vi "Dropable_DSA.vi"(0 "TF Out (CH B)":dbl, 1 "Cycle Specs":T2={"Cycles To Settle (M)"=5, "Cycles To Calculate (N)"=5}, 2 "Excitation Specs":T1={"Initial Frequency"=1.0, "Final Frequency"=100.0, "Number of Frequencies"=3, "Samping Time [s]"=0.001, "Amplitude [V]"=1.0, "Offset [V]"=0.5, "Freq Unit"=FALSE}, 5 "TF In (CH A)":dbl, 9 "START":bool, 11 "STOP":bool, 12 "Exist Porgram":bool) -> (4 "Disturbance":dbl, 6 "Bode Magnitude":cluster{dbl[], dbl[]}(graph)={[1.0, 1.2689610031679222, 1.6102620275609394, 2.043359717856942, 2.592943797404667, 3.2903445623126686, 4.1753189365604015, 5.298316906283708, 6.7233575364993365, 8.531678524172808, 10.826367338740546, 13.73823795883263, 17.43328822199988, 22.122162910704493, 28.072162039411772, 35.62247890262442, 45.20353656360243, 57.36152510448679, 72.7895384398315, 92.36708571873861, 117.21022975334806, 148.73521072935117, 188.73918221350976, 239.5026619987486, 303.9195382313198, 385.6620421163472, 489.3900918477494, 621.0169418915616, 788.0462815669912, 1000.0], [1.0018651131002922, 1.0016050465725763, 1.0010062349698785, 1.0002931137870483, 0.9991459144089636, 0.9972202532472595, 0.9944020144562293, 0.9903082002861369, 0.983855401702225, 0.9738705481650444, 0.9582906977613652, 0.9358034848813956, 0.9036393454169751, 0.857649976648417, 0.7964400088413218, 0.7217565791716765, 0.6359239660806931, 0.5476382842843324, 0.461415834347026, 0.38116988425483045, 0.3091314427820101, 0.2514928062528439, 0.20170891904461263, 0.15879614847289658, 0.127858110424497, 0.10171304349328705, 0.08081117825531599, 0.06376794604720305, 0.050469140870365095, 0.039745706120179934]}, 8 "Bode Phase":cluster{dbl[], dbl[]}(graph)={[1.0, 1.2689610031679222, 1.6102620275609394, 2.043359717856942, 2.592943797404667, 3.2903445623126686, 4.1753189365604015, 5.298316906283708, 6.7233575364993365, 8.531678524172808, 10.826367338740546, 13.73823795883263, 17.43328822199988, 22.122162910704493, 28.072162039411772, 35.62247890262442, 45.20353656360243, 57.36152510448679, 72.7895384398315, 92.36708571873861, 117.21022975334806, 148.73521072935117, 188.73918221350976, 239.5026619987486, 303.9195382313198, 385.6620421163472, 489.3900918477494, 621.0169418915616, 788.0462815669912, 1000.0], [-1.4001864556390353, -1.7425257743205063, -2.2774811113746067, -2.940300047591337, -3.797024621582645, -4.874740361894845, -6.244214499985965, -7.9488896703659435, -10.107416371370137, -12.8129960492024, -16.195047872218314, -20.2121008365249, -24.982209581081694, -30.62002310970157, -36.70295501035055, -43.18506539585506, -49.773026506300724, -56.0120451118291, -61.68921924132383, -66.61507141784128, -71.21117465500357, -75.07757805867544, -77.49128997241446, -81.82799122918105, -82.40583459630555, -84.09391534817092, -87.5421411007668, -88.23137376055858, -91.93060722680163, -98.46625820370649]}, 10 "Live Signals":cluster{"DSA Excitation":dbl, "output y(t)":dbl}(graph), 14 "Stopped":bool, 15 "Running":bool)   [LabVIEW 2017, in "DSA.lvlib"]
doc: "This program performs 3 tasks:\n\n A.) generates a swept sine wave over a specified number of logmartically spaced frequencies over a specified range,\n\n B.) outputs the swept sine wave point by point to a system and for each point output measues the system's response at two points\n\n C.) and using the two responses measured, calculates the bode magnitude and phase plots between the two points of the system.\n\nThis program is written as a state machine that itterates one time for every iteration of the loop that contains it.\n \nThe state is the current sample being measured. \nNOTE: Since we must excite the system before recording data, the current sample being measured is one less than the number of itterations the loop containing this subVI has run.\n\nTo perform these tasks, the following state machine does the following:\n\n INITIALIZATION \n\n When initalized, the state is set to 0 and the following are calculated:\n\n A.) a list of logmartically spaced frequencies to excite the system at, \n B.) the number of samples needed to be ignored in waiting for the excitation to settle for each frequency, \n C.) the number of samples needed to be measured in order to calculate the frequency response for each frequency,\n D.) and the total number of samples needed (total # of smaples ignored + total # of samples measured).\n\n < see (1) INITIALIZE THE DSA section in the block diagram >\n\n RUNNING\n\n When running, the following tasks are done:\n\n A.) The swept sine wave for the next sample to be measured is generated and output. \n This is done by generating:\n\n 1.) the ith point of the swept sine wave to excite the system\n 2.) the frequency of the sine wave for the current point\n 3.) and the index of the frequency within the list excitation frequencies that corresponds to the i+1 point's sine wave's frequency.\n\n < see (2A) GENERATE SWEPT SINE EXCITATIONS section in the block diagram >\n\n B.) Compare the current sample to:\n\n 1.) the current last sample to be ignored in the list of last samples to be ignored\n 2.) and the current last smaple taken before chaning frequencies in the list of sample taken before the frequency change.\n\n < see (2B) COLLECT DATA? section in the block diagram >\n\n C.) If the current sample:\n \n 1.) < the current last sample to be ignored:\n \n - do nothing.\n \n 2.) = the current last sample to be ignored and:\n\n\n a.) < the current sample taken before changing frequencies:\n \n - collect a sample on each channel and store it\n\n < see (2C) ANALYZE DATA section in the block diagram >\n\n b.) = the current sample taken before changing frequencies:\n\n i.) collect a sample on each channel and store it,\n ii.) with all the other samples stored for that excitation frequency, calculate the magnitude and phase for each channel,\n iii.) use the magnitude and phase for each channel to calculate the magnitude and phase between the two points in the system,\n iv.) and plot the magnitude and phase between those two points in the system on the bode plot for the frequency.\n \n < see (2D) VERIFY DATA & (2E) PLOT section in the block diagram >\n\nInputs: \n\n- Excitation Specs:\n\n - Initial Frequency: The lowest frequency of the frequency range which the DSA will measure the bode plot for. \n\n - Final Frequency: The highest frequency of the frequency range which the DSA will measure the bode plot for. \n\n - Frequency Units: Whether the frequecny range input is in Hz or rads/sec. \n \n - Number of Frequencies: The number of logmarithmically spaced frequencies to measure the bode plot for.\n\n - Sampling Time: The time step taking in between each measurement. Also equal to 1/(sampling rate)\n\n - Amplitude: Amplitude of desired swept sine excitation. \n\n - Offset: DC offset of swept sine excitation.\n\n- Cycle Specs:\n\n - Cycles to Settle: The number of cycles of the swept sine wave at each frequency to ignore to let the transcient response die out. \n\n - Cycles to Calculate: The number of cycles of the sept since wave at each frequency to measure in order to measure the bode plot.\n\n- Controls:\n\n - START: Tells the DSA to initalize and then start.\n\n - STOP: Tells the DSA to stop and set all analog outputs to zero.\n\n - EXIT PROGRAM: Tells LabVIEW to set all analog outputs to zero and exit the program.\n\n- Signals:\n\n - Analog In CH1: Response read by the A/D converter of the system at a given point to the swept sine excitation.\n\n - Analog In CH0: Response read by the A/D converter of the system at a given point to the swept sine excitation.\n\nOutputs:\n\n- Analog Out: Swept sine excitation wave sent to the D/A converter.\n\n- Running: Signal to show if the DSA is running.\n\n- Stopped: Signal to show if the DSA is stopped.\n\n- Bode Magnitude: The magnitude plot of the TF CH1/CH0.\n\n- Bode Phase: The phase plot of the TF CH1/CH0."
uses:
  DSA.lvlib
  <vilib>/Analysis/NI_AALPro.lvlib
panel:
  # "Dropable Dynamic Signal Analyzer"
  # "Magnitude"
  # "Dynamic Signal Analyzer"
  # "Controls"
  # "Signals"
  # "Phase"
  # "Excitation Frequencies"
  # "Frequency\nUnits"
  # "[Hz]"
  # "Excitation Magnitude"
  # "[rad/s]"
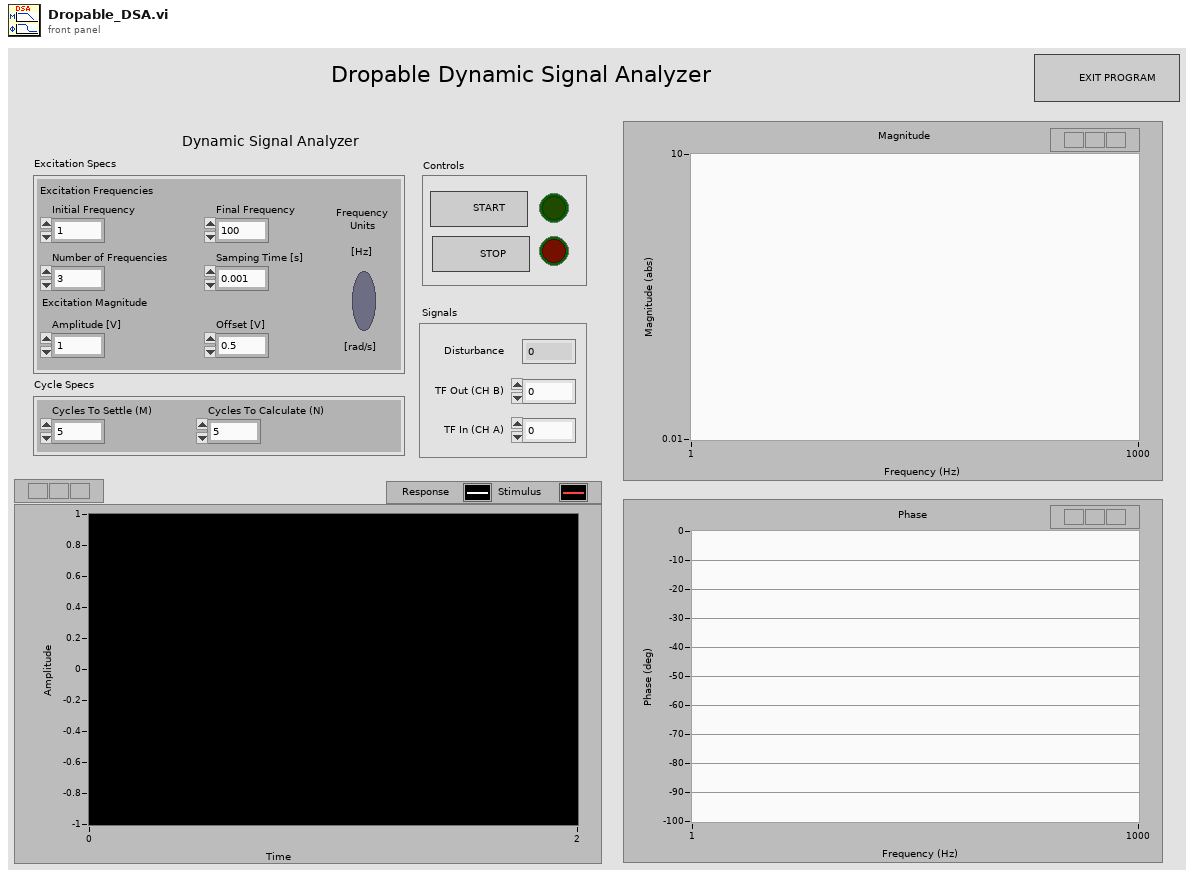
[diagram p1: front panel]
types:
  T1 = cluster{"Initial Frequency":dbl, "Final Frequency":dbl, "Number of Frequencies":i16, "Samping Time [s]":dbl, "Amplitude [V]":dbl, "Offset [V]":dbl, "Freq Unit":bool}
  T2 = cluster{"Cycles To Settle (M)":i16, "Cycles To Calculate (N)":i16}
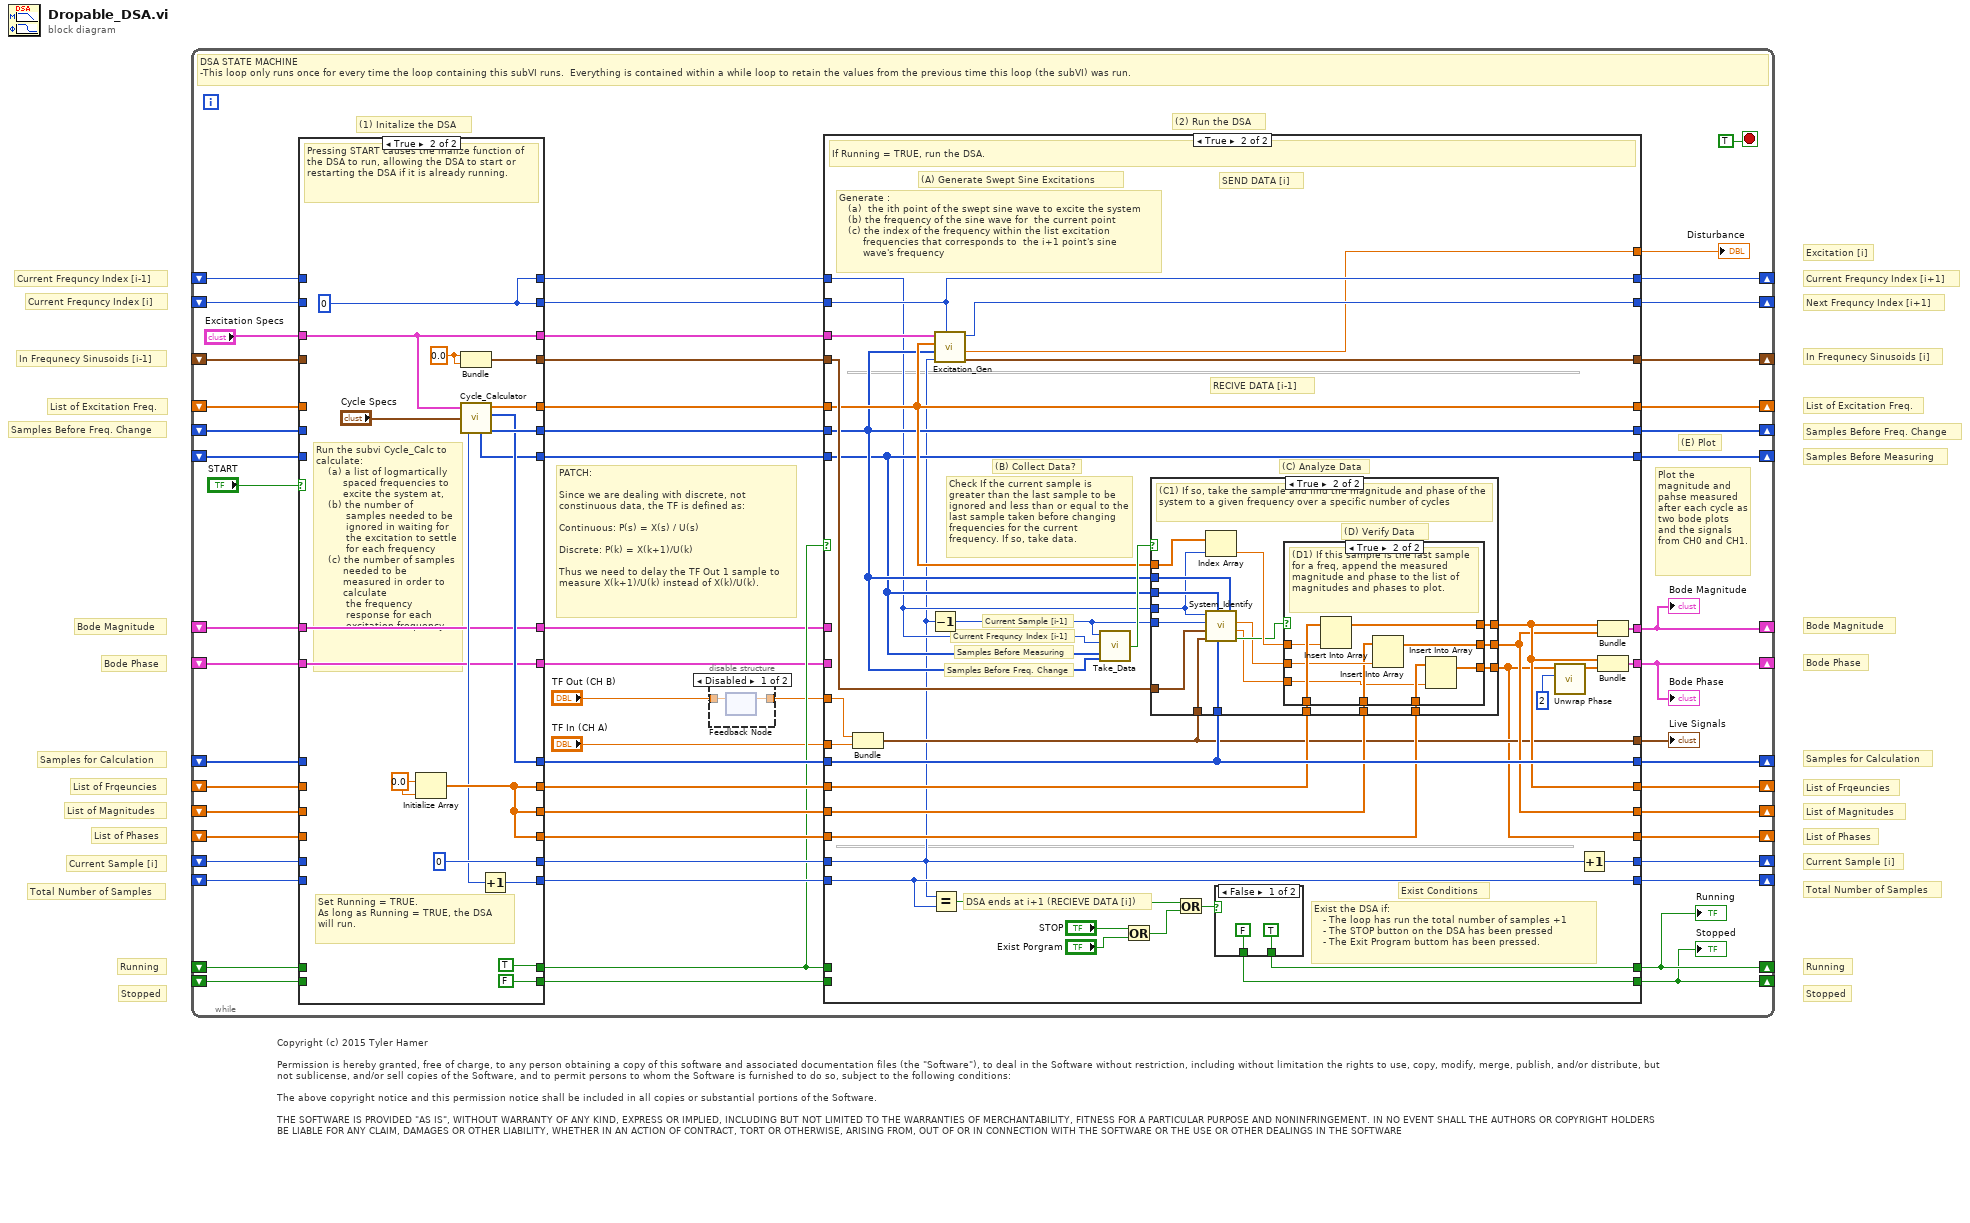
[diagram p0: block diagram]
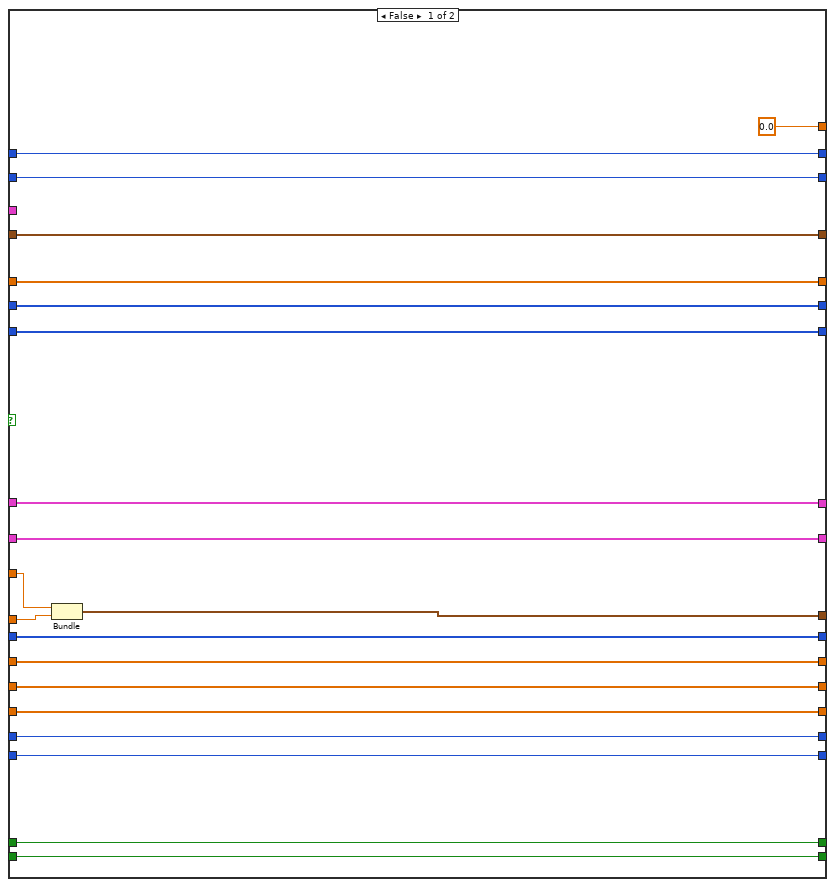
[diagram p4: hidden frame]
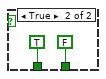
[diagram p5: hidden frame]
diagram:
  # "Copyright (c) 2015 Tyler Hamer\n\nPermission is hereby granted, free of charge, to any person obtaining a copy of this software and associated documentation files (the \"Software\"), to deal in the Software without restriction, including without limitation the rights to use, copy, modify, merge, publish, and/or distribute, but not sublicense, and/or sell copies of the Software, and to permit persons to whom the Software is furnished to do so, subject to the following conditions:\n\nThe above copyright notice and this permission notice shall be included in all copies or substantial portions of the Software.\n\nTHE SOFTWARE IS PROVIDED \"AS IS\", WITHOUT WARRANTY OF ANY KIND, EXPRESS OR IMPLIED, INCLUDING BUT NOT LIMITED TO THE WARRANTIES OF MERCHANTABILITY, FITNESS FOR A PARTICULAR PURPOSE AND NONINFRINGEMENT. IN NO EVENT SHALL THE AUTHORS OR COPYRIGHT HOLDERS BE LIABLE FOR ANY CLAIM, DAMAGES OR OTHER LIABILITY, WHETHER IN AN ACTION OF CONTRACT, TORT OR OTHERWISE, ARISING FROM, OUT OF OR IN CONNECTION WITH THE SOFTWARE OR THE USE OR OTHER DEALINGS IN THE SOFTWARE"
  # "Bode Phase"
  # "Bode Magnitude"
  # "Bode Phase"
  # "Bode Magnitude"
  # "Stopped"
  # "Running"
  # "Stopped"
  # "Running"
  # "Total Number of Samples"
  # "Total Number of Samples"
  # "List of Phases"
  # "List of Magnitudes"
  # "List of Frqeuncies"
  # "List of Phases"
  # "List of Magnitudes"
  # "List of Frqeuncies"
  # "Samples Before Measuring"
  # "Samples Before Freq. Change"
  # "Current Sample [i]"
  # "Samples for Calculation"
  # "Excitation [i]"
  # "List of Excitation Freq."
  # "In Frequnecy Sinusoids [i]"
  # "Next Frequncy Index [i+1]"
  # "Current Frequncy Index [i+1]"
  # "Samples for Calculation"
  # "Current Sample [i]"
  # "Samples Before Freq. Change"
  # "In Frequnecy Sinusoids [i-1]"
  # "Current Frequncy Index [i-1]"
  # "Current Frequncy Index [i]"
  # "List of Excitation Freq."
  n1 = while {
    shift-right: [w49] -> _
    shift-left: _ -> [w53]
    shift-right: [w51] -> _
    shift-left: _ -> [w52]
    shift-right: [w47] -> _
    shift-left: _ -> [w46]
    shift-right: [w40] -> _
    shift-left: _ -> [w50]
    shift-right: [w44] -> _
    shift-left: _ -> [w43]
    shift-right: [w37] -> _
    shift-left: _ -> [w36]
    shift-right: [w34] -> _
    shift-left: _ -> [w33]
    shift-right: [w31] -> _
    shift-left: _ -> [w30]
    shift-right: [w23] -> _
    shift-left: _ -> [w26]
    shift-right: [w22] -> _
    shift-left: _ -> [w25]
    shift-right: [w21] -> _
    shift-left: _ -> [w24]
    shift-right: [w18] -> _
    shift-left: _ -> [w17]
    shift-right: [w12] -> _
    shift-left: _ -> [w16]
    shift-right: [w11] -> _
    shift-left: _ -> [w13]
    shift-right: [w5] -> _
    shift-left: _ -> [w10]
    shift-right: [w4] -> _
    shift-left: _ -> [w9]
    stop <- TRUE stop-if-true
    # "PATCH:\n \nSince we are dealing with discrete, not constinuous data, the TF is defined as:\n \nContinuous: P(s) = X(s) / U(s) \n \nDiscrete: P(k) = X(k+1)/U(k)\n \nThus we need to delay the TF Out 1 sample to measure X(k+1)/U(k) instead of X(k)/U(k)."
    # "Plot the magnitude and pahse measured after each cycle as two bode plots and the signals from CH0 and CH1."
    # "(E) Plot"
    # "(2) Run the DSA"
    # "(1) Initalize the DSA"
    # "DSA STATE MACHINE \n-This loop only runs once for every time the loop containing this subVI runs.  Everything is contained within a while loop to retain the values from the previous time this loop (the subVI) was run."
    n2 = case shown="True" "START" {
      tunnel: "Excitation Specs" -> [w77 w94]
      tunnel: [w77 w94] -> w55
      tunnel: [w75 w93] -> w54
      tunnel: w53 -> [w75 _]
      tunnel: [w76 w91] -> w48
      tunnel: w52 -> [w76 _]
      tunnel: [w72 w92] -> w41
      tunnel: w50 -> [w72 _]
      tunnel: [w74 w91] -> w45
      tunnel: w46 -> [w74 _]
      tunnel: w43 -> [w73 _]
      tunnel: [w73 w89] -> w42
      tunnel: [w71 0] -> w39
      tunnel: w36 -> [w71 _]
      tunnel: [w70 w87] -> w35
      tunnel: w33 -> [w70 _]
      tunnel: [w69 w86] -> w32
      tunnel: w30 -> [w69 _]
      tunnel: [w68 w84] -> w29
      tunnel: [w67 w84] -> w28
      tunnel: [w66 w84] -> w27
      tunnel: w26 -> [w68 _]
      tunnel: w25 -> [w67 _]
      tunnel: w24 -> [w66 _]
      tunnel: [w65 w81] -> w19
      tunnel: w17 -> [w65 _]
      tunnel: w16 -> [w64 _]
      tunnel: [w64 TRUE] -> w15
      tunnel: [w63 FALSE] -> w14
      tunnel: w13 -> [w63 _]
      tunnel: w10 -> [w62 w79]
      tunnel: w9 -> [w61 w78]
      tunnel: [w62 w79] -> w8
      tunnel: [w61 w78] -> w7
      frame False {
      }
      frame True {
        w85 = 0.0
        w90 = 0.0
        w91 = 0
        # "Run the subvi Cycle_Calc to calculate: \n    (a) a list of logmartically \n         spaced frequencies to \n         excite the system at, \n    (b) the number of \n          samples needed to be \n          ignored in waiting for \n          the excitation to settle \n          for each frequency \n    (c) the number of samples \n         needed to be \n         measured in order to\n         calculate \n          the frequency   \n          response for each \n          excitation frequency."
        # "Set Running = TRUE.\nAs long as Running = TRUE, the DSA\nwill run."
        # "Pressing START causes the inalize function of the DSA to run, allowing the DSA to start or restarting the DSA if it is already running."
        n3 = Initialize Array(w85, w85) -> (w84:dbl[])
        n4 = Bundle(w90, w90) -> (w89:cluster{dbl, dbl})  [unwired: 1 in]
        n5 = call "Cycle_Calculator.vi"("Cycle Specs"="Cycle Specs", "Excitation Specs"=w94) -> ("Samples Before Frequency Change"=w92:i32[], "Samples Before Measuring"=w86:i32[], "Samples for Calculation"=w87:i32[], "Excitation Frequencies"=w93:dbl[], "Total Number of Samples"=w80:i32)  [unwired: 1 in, 1 out]
        n6 = Increment(x=w80) -> (x+1=w81:i32)
      }
    }
    n7 = disable-structure shown="Disabled" {
      disable-tunnel: "TF Out (CH B)" -> [w59 w60]
      disable-tunnel: [w58 w60] -> w2
      frame Disabled {
        n8 = feedback #1() -> (w58:dbl)  [unwired: 1 in]
        n9 = feedback-in #1(w59) -> ()
      }
      frame Enabled {
      }
    }
    n10 = case shown="True" w15 {
      tunnel: w55 -> [_ w151]
      tunnel: w54 -> [w115 w144]
      tunnel: [w114 w150] -> w51
      tunnel: [w115 w144] -> w49
      tunnel: w48 -> [w114 w149]
      tunnel: [w113 w149] -> w47
      tunnel: w45 -> [w113 w141]
      tunnel: [w112 w148] -> w44
      tunnel: w42 -> [w112 w145]
      tunnel: w41 -> [w111 w143]
      tunnel: [w111 w143] -> w40
      tunnel: w39 -> [w110 w119]
      tunnel: [w110 w147] -> w37
      tunnel: w35 -> [w109 w137]
      tunnel: [w109 w137] -> w34
      tunnel: w32 -> [w108 w142]
      tunnel: [w108 w142] -> w31
      tunnel: w2 -> [w99 w139]
      tunnel: "TF In (CH A)" -> [w98 w138]
      tunnel: w29 -> [w107 w136]
      tunnel: w28 -> [w106 w135]
      tunnel: w27 -> [w105 w134]
      tunnel: [w107 w133] -> w23
      tunnel: [w106 w132] -> w22
      tunnel: [w105 w118] -> w21
      tunnel: [0.0 w131] -> w20
      tunnel: w19 -> [w104 w123]
      tunnel: [w104 w123] -> w18
      tunnel: w15 -> [w103 _]
      tunnel: [w103 w125] -> w12
      tunnel: [w102 w124] -> w11
      tunnel: w14 -> [w102 _]
      tunnel: [w101 w121] -> w5
      tunnel: [w100 w120] -> w4
      tunnel: w8 -> [w101 _]
      tunnel: w7 -> [w100 _]
      tunnel: [w97 w122] -> w6
      frame False {
        n11 = Bundle("TF Out (CH B)"=w99, "TF In (CH A)"=w98) -> (w97:cluster{"TF Out (CH B)":dbl, "TF In (CH A)":dbl})  [unwired: 1 in]
      }
      frame True {
        # "(C) Analyze Data"
        # "Exist Conditions"
        # "Exist the DSA if:\n   - The loop has run the total number of samples +1\n   - The STOP button on the DSA has been pressed\n   - The Exit Program buttom has been pressed."
        # "DSA ends at i+1 (RECIEVE DATA [i])"
        # "SEND DATA [i]"
        # "RECIVE DATA [i-1]"
        # "Samples Before Freq. Change"
        # "Samples Before Measuring"
        # "Current Frequncy Index [i-1]"
        # "Current Sample [i-1]"
        # "(B) Collect Data?"
        # "Check If the current sample is greater than the last sample to be ignored and less than or equal to the last sample taken before changing frequencies for the current frequency. If so, take data."
        # "(A) Generate Swept Sine Excitations"
        # "Generate :\n   (a)  the ith point of the swept sine wave to excite the system\n   (b) the frequency of the sine wave for  the current point\n   (c) the index of the frequency within the list excitation \n        frequencies that corresponds to  the i+1 point's sine \n        wave's frequency"
        # "If Running = TRUE, run the DSA."
        n12 = Bundle("TF Out (CH B)"=w139, "TF In (CH A)"=w138) -> (w122:cluster{"TF Out (CH B)":dbl, "TF In (CH A)":dbl})  [unwired: 1 in]
        n13 = Decrement(x=w119) -> (x-1=w140:i32)
        n14 = Equal?(x=w119, y=w123) -> (x = y?=w130:bool)
        n15 = call "Excitation_Gen.vi"("Current Frequency Index"=w149, "Current Sample"=w119, "Samples Before Frequency Change"=w143, "Excitation Frequencies"=w144, "Excitation Specs"=w151) -> ("In Frequency Sinusoids"=w148:cluster{"cos(wt)":dbl, " sin(wt)":dbl}, "Excitation Sinusoid"=w131:dbl, "New Frequency Index"=w150:i32)  [unwired: 1 out]
        n16 = call "Take_Data.vi"("Samples Before Frequency Change"=w143, "Samples Before Measuring"=w142, "Current Frequency Index"=w141, "Current Sample"=w140) -> ("Take Data"=w146:bool)
        n17 = Or(x="STOP", y="Exist Porgram") -> (x .or. y?=w127:bool)
        n18 = case shown="True" w146 {
          tunnel: w145 -> [_ w172]
          tunnel: w122 -> [_ w176]
          tunnel: w140 -> [_ w175]
          tunnel: w141 -> [_ w169]
          tunnel: w142 -> [_ w174]
          tunnel: w143 -> [_ w173]
          tunnel: w144 -> [_ w171]
          tunnel: w137 -> [_ w170]
          tunnel: w136 -> [w158 w164]
          tunnel: w135 -> [w157 w163]
          tunnel: w134 -> [w156 w162]
          tunnel: [w158 w161] -> w133
          tunnel: [w157 w160] -> w132
          tunnel: [w156 w159] -> w118
          frame False {
            # "(C2) If not, ignore the current samples. Pass throught the list of measured magnitude and phases though."
          }
          frame True {
            # "(D) Verify Data"
            # "(C1) If so, take the sample and find the magnitude and phase of the system to a given frequency over a specific number of cycles"
            n19 = Index Array(array=w171, index=w169) -> (element=w168:dbl)
            n20 = call "System_Identify.vi"("Samples Before Frequency Change"=w173, "Samples for Calculation"=w170, "Samples Before Measuring"=w174, "Frequency Responses"=w176, "In Frequency Sinusoids"=w172, "Current Sample"=w175, "Current Frequency Index"=w169) -> ("Push To Plot"=w167:bool, "System Phase"=w165:dbl, "System Magnitude"=w166:dbl)
            n21 = case shown="True" w167 {
              tunnel: w168 -> [_ w187]
              tunnel: w166 -> [_ w186]
              tunnel: w165 -> [_ w183]
              tunnel: w164 -> [w179 w188]
              tunnel: w163 -> [w178 w185]
              tunnel: w162 -> [w177 w184]
              tunnel: [w179 w182] -> w161
              tunnel: [w178 w181] -> w160
              tunnel: [w177 w180] -> w159
              frame False {
                # "(D2) If this sample is not the last sample for a freq, the current measured magnitude and phase are not accurate yet."
              }
              frame True {
                # "(D1) If this sample is the last sample for a freq, append the measured magnitude and phase to the list of magnitudes and phases to plot."
                n22 = Insert Into Array(array=w188, new element=w187) -> (w182:dbl[])  [unwired: 1 in]
                n23 = Insert Into Array(array=w185, new element=w186) -> (w181:dbl[])  [unwired: 1 in]
                n24 = Insert Into Array(array=w184, new element=w183) -> (w180:dbl[])  [unwired: 1 in]
              }
            }
          }
        }
        n25 = Or(x=w130, y=w127) -> (x .or. y?=w126:bool)
        n26 = case shown="False" w126 {
          tunnel: [TRUE FALSE] -> w125
          tunnel: [FALSE TRUE] -> w124
          frame False {
          }
          frame True {
          }
        }
        n27 = call <vilib>:"Unwrap Phase.vi"("phase unit"=2, "Phase"=w118) -> ("Unwrapped Phase"=w117:dbl[])  [unwired: 8 in, 1 out]
        n28 = Increment(x=w119) -> (x+1=w147:i32)
        n29 = Bundle(w133, w132) -> (w121:cluster{dbl[], dbl[]})  [unwired: 1 in]
        n30 = Bundle(w133, "Unwrapped Phase"=w117) -> (w120:cluster{dbl[], "Unwrapped Phase":dbl[]})  [unwired: 1 in]
      }
    }
    "Disturbance" <- w20
    "Running" <- w12
    "Stopped" <- w11
    "Live Signals" <- w6
    "Bode Magnitude" <- w5
    "Bode Phase" <- w4
  }
